vi "EOL CAN_Write Vehicle Type.vi"(10 "Read Session in":refnum<k21>, 11 "Write Session in":refnum<k21>) -> (0 "error out":errorcluster, 1 "Rx Message":u8[](array[numeric]), 2 "Response Good?":bool, 3 "Array":string[][](array[string]))   [LabVIEW 2018]
uses:
  <vilib>/xnet/xnet.llb/XNET Frame CAN.ctl
  <vilib>/xnet/xnet.llb/XNET Frame Type CAN.ctl
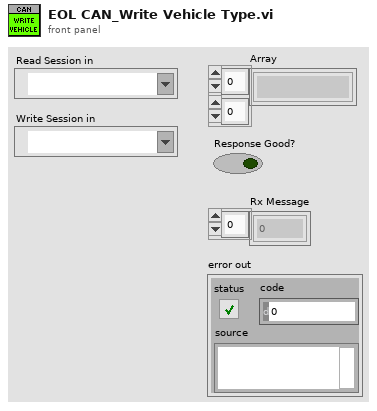
[diagram p1: front panel]
types:
  T1 = typedef "XNET Frame CAN.ctl" = cluster{"timestamp":timestamp, "payload":u8[], "identifier":u32, "type":T2, "extended?":bool, "echo?":bool}
  T2 = typedef "XNET Frame Type CAN.ctl" = u8
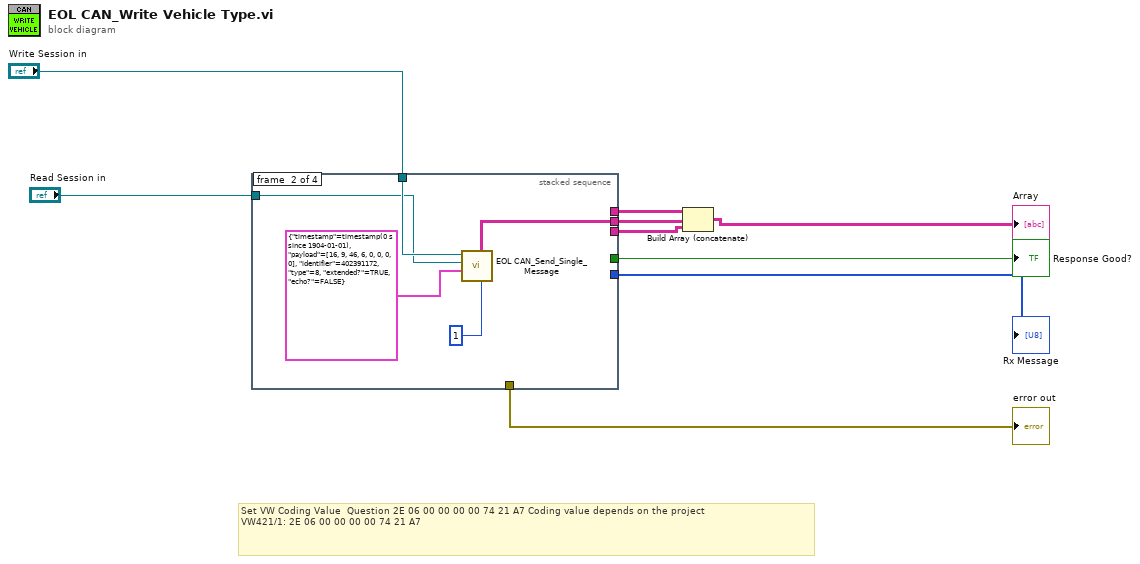
[diagram p0: block diagram]
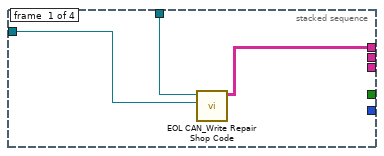
[diagram p2: hidden frame]
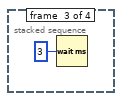
[diagram p3: hidden frame]
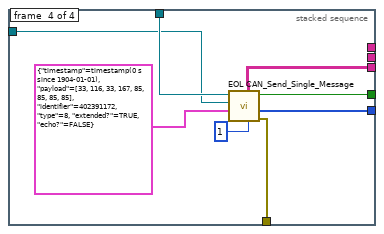
[diagram p4: hidden frame]
diagram:
  # "Set VW Coding Value \tQuestion\t2E 06 00 00 00 00 74 21 A7\tCoding value depends on the project\nVW421/1: 2E 06 00 00 00 00 74 21 A7"
  n1 = stacked-sequence {
    tunnel: "Write Session in" -> [w12 w17 _ w26]
    tunnel: "Read Session in" -> [w11 w16 _ w25]
    tunnel: [_ _ _ w20] -> w4
    tunnel: [_ _ _ w23] -> w5
    tunnel: [_ _ _ w21] -> w6
    tunnel: [w10 _ _ _] -> w7
    tunnel: [_ w13 _ _] -> w8
    tunnel: [_ _ _ w19] -> w9
    frame #0 {
      n2 = call "EOL CAN_Write Repair Shop Code.vi"("Read Session in"=w11, "Write Session in"=w12) -> ("TxRxData"=w10:string[][])  [unwired: 6 in, 3 out]
    }
    frame #1 {
      n3 = call "EOL CAN_Send_Single_Message.vi"("Retries"=1, "Tx CAN frame"=T1 {"timestamp"=timestamp(0 s since 1904-01-01), "payload"=[16, 9, 46, 6, 0, 0, 0, 0], "identifier"=402391172, "type"=8, "extended?"=TRUE, "echo?"=FALSE}, "Read Session in"=w16, "Write Session in"=w17) -> ("TxRx Data"=w13:string[][])  [unwired: 3 in, 4 out]
    }
    frame #2 {
      n4 = Wait (ms)(milliseconds to wait=u32 3) -> ()  [unwired: 1 out]
    }
    frame #3 {
      n5 = call "EOL CAN_Send_Single_Message.vi"("Retries"=1, "Tx CAN frame"=T1 {"timestamp"=timestamp(0 s since 1904-01-01), "payload"=[33, 116, 33, 167, 85, 85, 85, 85], "identifier"=402391172, "type"=8, "extended?"=TRUE, "echo?"=FALSE}, "Read Session in"=w25, "Write Session in"=w26) -> ("Error out"=w20:errorcluster, "Rx Message"=w21:u8[], "Response Good?"=w23:bool, "TxRx Data"=w19:string[][])  [unwired: 3 in, 1 out]
    }
  }
  "Rx Message" <- w6
  "Response Good?" <- w5
  "error out" <- w4
  n6 = Build Array (concatenate)(w7, w8, w9) -> (→"Array":string[][])
